vi "Init.vi"(8 "error in (no error)":errorcluster, 9 "Data":variant, 10 "Type":i32) -> (0 "error out":errorcluster, 3 "VariantMessage out":refnum<class "VariantMessage.lvclass">)   [LabVIEW 2013, in "VariantMessage.lvclass"]
doc: "Initializes a message with type and data"
uses:
  VariantMessage.lvclass
  VariantMessage.lvclass/VariantMessage.ctl
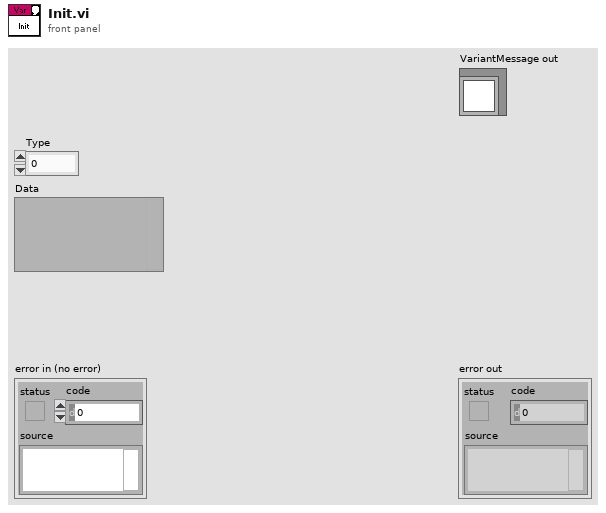
[diagram p1: front panel]
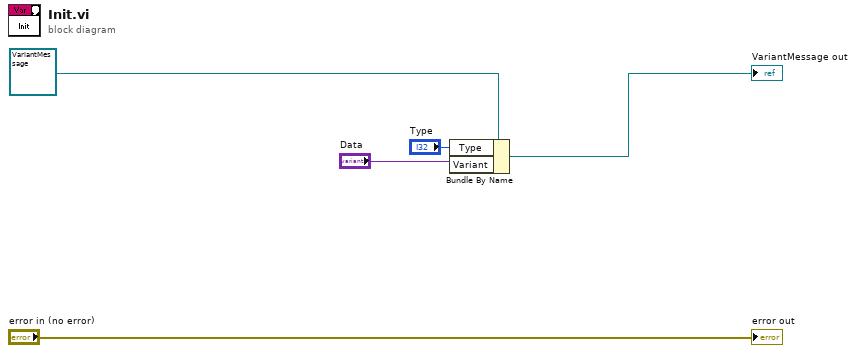
[diagram p0: block diagram]
diagram:
  n1 = Bundle By Name(cluster=refnum<class "VariantMessage.lvclass"> refnum ("VariantMessage.lvclass"), "Type"="Type", "Variant"="Data") -> (→"VariantMessage out":refnum<class "VariantMessage.lvclass">)
  "error out" <- "error in (no error)"
